vi "TranslateVirtualStave.vi"(5 "Tooling Pin Orientation":bool=TRUE, 6 "ZStopToCalibrationOrigin":dbl[](array[numeric])=[19.434, 9.7121] format="%#_10g", 7 "Stave Orientation":bool=TRUE, 8 "error in":errorcluster, 9 "Angle between stave and xyz stage":dbl=0.0006396233435161352, 10 "Calibrated stave origin (X,Y) [mm]":dbl[](array[numeric])=[570.2627012368548, -37.200267571549986], 11 "Stave Basis: Coordinates of Fiducials on Modules":dbl[][](array[numeric])) -> (0 "Error out":errorcluster[](array[cluster]), 3 "Virtual Stave":dbl[][](array[numeric]))   [LabVIEW 2016]
uses:
  <vilib>/Analysis/coordinate.llb/2D Cartesian Coordinate Shift (Scalar).vi
  <vilib>/Analysis/NI_AALPro.lvlib
panel:
  out "dx origin":dbl
  out "dy origin":dbl
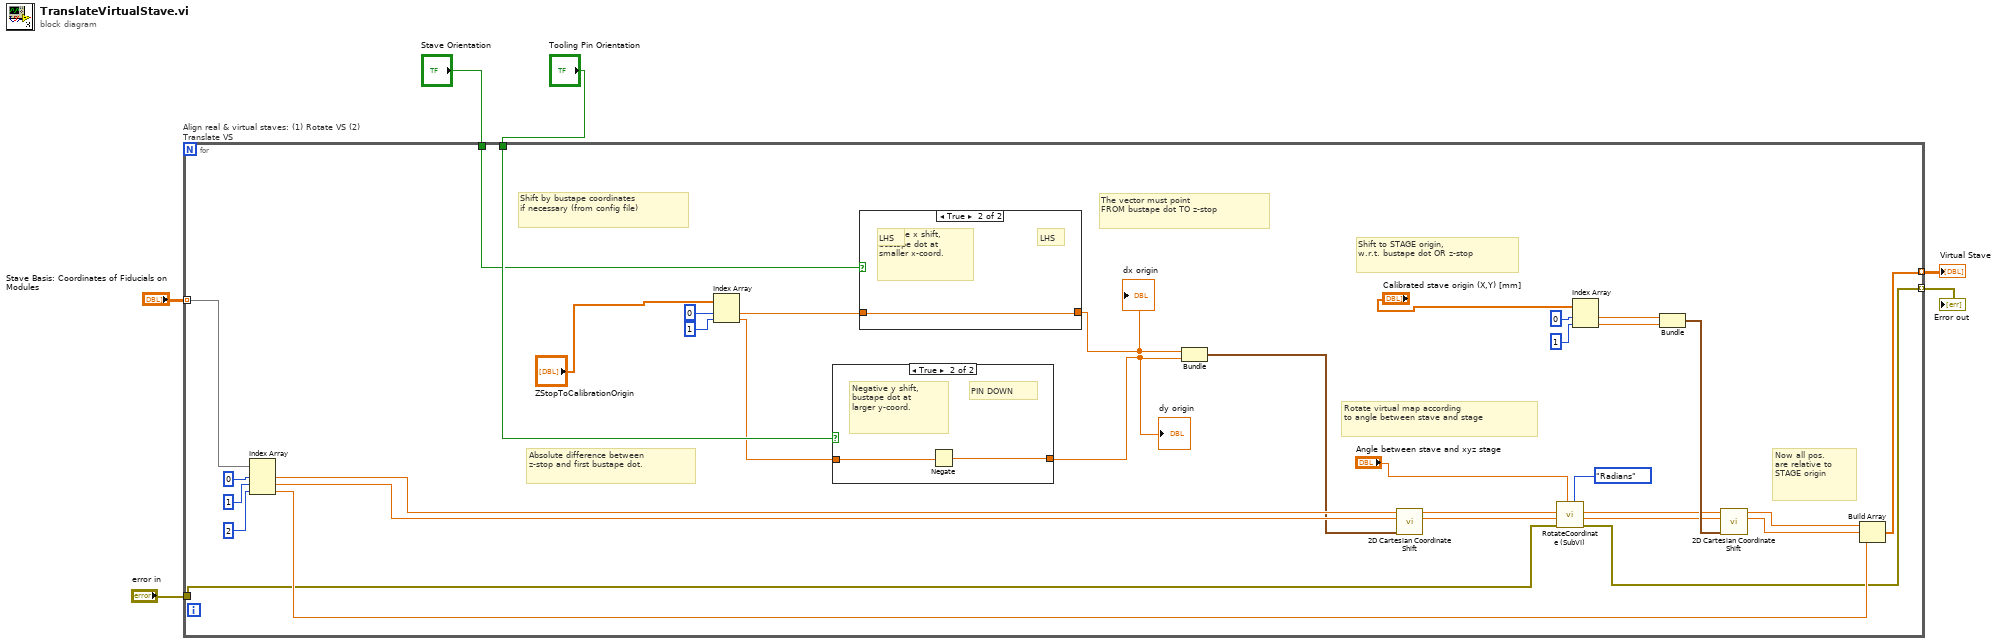
[diagram p0: block diagram]
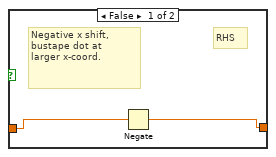
[diagram p3: hidden frame]
diagram:
  n1 = for "Align real & virtual staves: (1) Rotate VS (2) Translate VS" {
    tunnel: "Stave Basis: Coordinates of Fiducials on Modules" -> [w31] mode=indexing
    tunnel: [w38] -> w4 mode=indexing
    tunnel: "error in" -> [w23]
    tunnel: [w24] -> w3 mode=indexing
    tunnel: "Tooling Pin Orientation" -> [w18]
    tunnel: "Stave Orientation" -> [w17]
    # "The vector must point \nFROM bustape dot TO z-stop"
    # "Absolute difference between\nz-stop and first bustape dot."
    # "Shift by bustape coordinates\nif necessary (from config file)"
    # "Now all pos.\nare relative to\nSTAGE origin"
    # "Shift to STAGE origin,\nw.r.t. bustape dot OR z-stop"
    # "Rotate virtual map according\nto angle between stave and stage"
    n2 = Index Array(array=w31, index #1=0 ("index"), index #2=1 ("index"), index #3=2 ("index")) -> (element #1=w20:dbl, element #2=w19:dbl, element #3=w34:dbl)
    n3 = Index Array(array="ZStopToCalibrationOrigin", index #1=0 ("index"), index #2=1 ("index")) -> (element #1=w13:dbl, element #2=w12:dbl)
    n4 = case shown="True" w18 {
      tunnel: w12 -> [w41 w43]
      tunnel: [w41 w42] -> w10
      frame False {
        # "PIN UP"
        # "Postive y shift, \nbustape dot at\nsmaller y-coord."
        # "PIN UP"
      }
      frame True {
        # "Negative y shift, \nbustape dot at\nlarger y-coord."
        # "PIN DOWN"
        n5 = Negate(x=w43) -> (-x=w42:dbl)
      }
    }
    "dy origin" <- w10
    n6 = case shown="True" w17 {
      tunnel: w13 -> [w45 w46]
      tunnel: [w44 w46] -> w11
      frame False {
        # "Negative x shift,\nbustape dot at \nlarger x-coord."
        # "RHS"
        n7 = Negate(x=w45) -> (-x=w44:dbl)
      }
      frame True {
        # "LHS"
        # "Positive x shift,\nbustape dot at \nsmaller x-coord."
        # "LHS"
      }
    }
    "dx origin" <- w11
    n8 = Bundle(w11, w10) -> (w16:cluster{dbl, dbl})  [unwired: 1 in]
    n9 = call-poly <vilib>:"2D Cartesian Coordinate Shift.vi"("shift"=w16, "y"=w19, "x"=w20) -> ("y out"=w22:dbl, "x out"=w21:dbl)  [unwired: 6 in, 1 out]
    n10 = call "RotateCoordinate (SubVI).vi"("Units"=enum16{"mrad", "Radians", "Degrees"}."Radians", "Angle"="Angle between stave and xyz stage", "error in (no error)"=w23, "y"=w22, "x"=w21) -> ("error out"=w24:errorcluster, "y'"=w27:dbl, "x'"=w26:dbl)  [unwired: 4 in]
    n11 = Index Array(array="Calibrated stave origin (X,Y) [mm]", index #1=0 ("index"), index #2=1 ("index")) -> (element #1=w33:dbl, element #2=w32:dbl)
    n12 = Bundle(w33, w32) -> (w28:cluster{dbl, dbl})  [unwired: 1 in]
    n13 = call-poly <vilib>:"2D Cartesian Coordinate Shift.vi"("shift"=w28, "y"=w27, "x"=w26) -> ("y out"=w30:dbl, "x out"=w29:dbl)  [unwired: 6 in, 1 out]
    n14 = Build Array(w29, w30, w34) -> (w38:dbl[])
  }
  "Virtual Stave" <- w4
  "Error out" <- w3
